vi "Read Module Configuration.vi"(8 "error in":errorcluster, 11 "slsc module":refnum<k21>) -> (0 "error out":errorcluster, 1 "switches json":string, 2 "topologies":string[](array[string]), 3 "product name":string, 4 "slot number":u32)   [LabVIEW 2020, in "SLSC Switch Scripting.lvlib"]
uses:
  SLSC Switch Scripting.lvlib
  <vilib>/SLSC_Switch/Get Topologies (Simulate).vi
  <vilib>/SLSC_Switch/SLSC Switch.lvlib
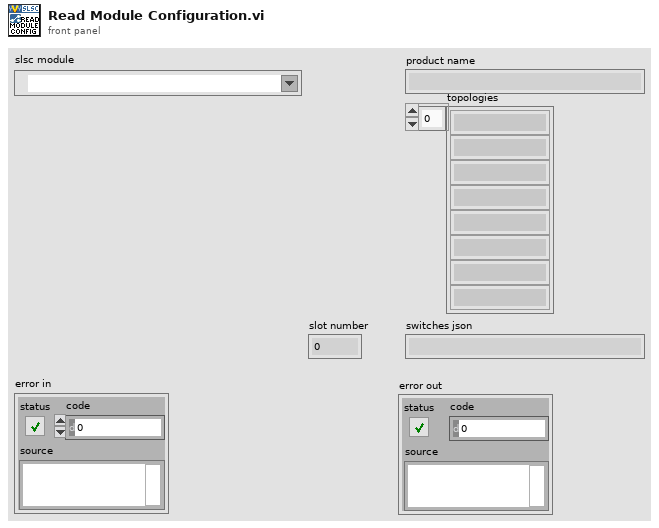
[diagram p1: front panel]
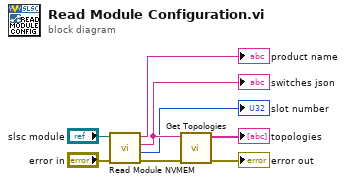
[diagram p0: block diagram]
diagram:
  n1 = call "Read Module NVMEM.vi"("error in"="error in", "slsc module"="slsc module") -> ("error out"=w4:errorcluster, "slot number"=→"slot number":u32, "switches json"=w2:string, "product name"=→"product name":string)  [unwired: 6 in]
  "switches json" <- w2
  n2 = call-poly <vilib>:"Get Topologies.vi"("error in (no error)"=w4, "switches json"=w2) -> ("error out"=→"error out":errorcluster, "topologies"=→"topologies":string[])  [unwired: 8 in]
